vi "CleanUp.vi"(8 "Error In":errorcluster, 11 "object in":refnum<class "Base1.lvclass">) -> (0 "Error Out":errorcluster, 3 "object out":refnum<class "Base1.lvclass">)   [LabVIEW 2020, in "RootLibrary.lvlib" / "Base1Library.lvlib" / "Base1.lvclass"]
uses:
  Base1.lvclass
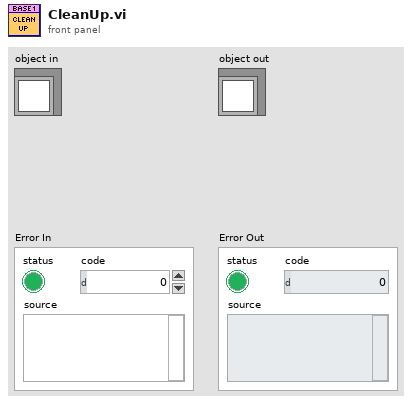
[diagram p1: front panel]
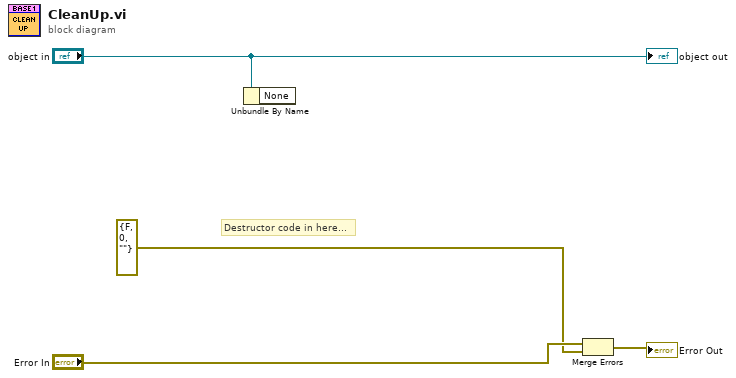
[diagram p0: block diagram]
diagram:
  # "Destructor code in here..."
  n1 = Unbundle By Name("object in") -> ()  [unwired: 1 out]
  n2 = Merge Errors("Error In", errorcluster {"status"=FALSE, "code"=0, "source"=""} ("error in (no error)")) -> (→"Error Out":errorcluster)
  "object out" <- "object in"
